vi "HexToFloat.vi"(7 "转换类型":enum16{"DCBA", "CDAB"}(ring), 11 "数组":u16[](array[numeric]) format="%04xH") -> (3 "FLOAT":sgl[](array[numeric]))   [LabVIEW 2016, in "质控单元V1.lvlib"]
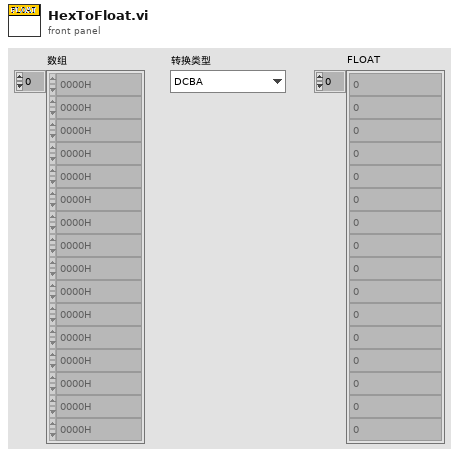
[diagram p1: front panel]
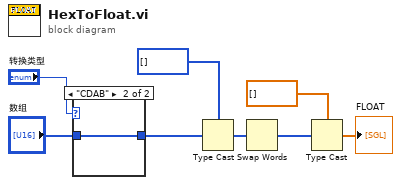
[diagram p0: block diagram]
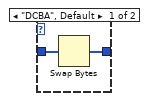
[diagram p2: hidden frame]
diagram:
  n1 = case shown="\"CDAB\"" "转换类型" {
    tunnel: "数组" -> [w10 w11]
    tunnel: [w9 w11] -> w2
    frame "DCBA", Default {
      n2 = Swap Bytes(anything=w10) -> (byte swapped=w9:u16[])
    }
    frame "CDAB" {
    }
  }
  n3 = Type Cast(type=u32[] [], x=w2) -> (*(type *) &x=w5:u32[])
  n4 = Swap Words(1:w5) -> (0:w4:u32[])
  n5 = Type Cast(type=sgl[] [], x=w4) -> (*(type *) &x=→"FLOAT":sgl[])
